vi "Retentive timer on（tool).vi"(8 "errorin":errorcluster caption="error in", 9 "reset":bool, 10 "preset time":u32=1000, 11 "enable":bool) -> (0 "error out":errorcluster, 2 "accumulated time":u32, 3 "done":bool)   [LabVIEW 2013, in "毫秒定时器.lvlib"]
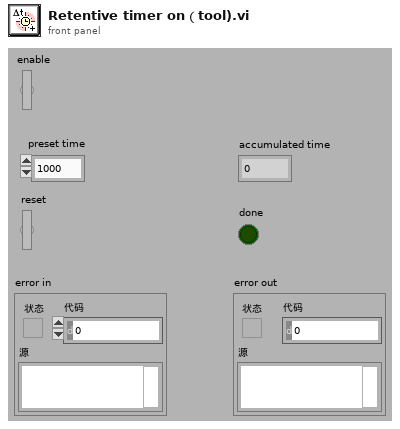
[diagram p1: front panel]
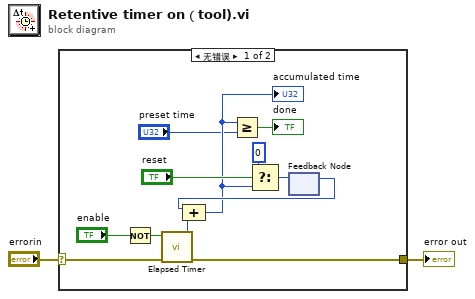
[diagram p0: block diagram]
diagram:
  n1 = case shown="无错误" "errorin" {
    selector: "errorin" -> [w4 w15]
    tunnel: [w3 w15] -> w1
    frame No Error {
      n2 = Not(x="enable") -> (.not. x?=w11:bool)
      n3 = call "Elapsed Timer.vi"("error in"=w4, "reset"=w11) -> ("error out"=w3:errorcluster, "since last call"=w13:u32)  [unwired: 7 in, 1 out]
      n4 = feedback #1() -> (w14:u32)  [unwired: 1 in]
      n5 = Compound Arithmetic op=ADD(w14, w13) -> (w7:u32)
      "accumulated time" <- w7
      n6 = Greater Or Equal?(x=w7, y="preset time") -> (x >= y?=→"done":bool)
      n7 = Select(t=u32 0 ("accumulated time"), s="reset", f=w7) -> (s? t:f=w8:u32)
      n8 = feedback-in #1(w8) -> ()
    }
    frame Error {
    }
  }
  "error out" <- w1
